vi "RWAE-Fix Name.vi"(8 "error in (no error)":errorcluster, 9 "Section Name (Name of \"Anything\")":string, 10 "Cluster Elements in":variant[](array[variant])) -> (0 "error out":errorcluster, 3 "Name":string)   [LabVIEW 2020]
uses:
  <vilib>/Utility/Data Type/NI_Data Type.lvlib
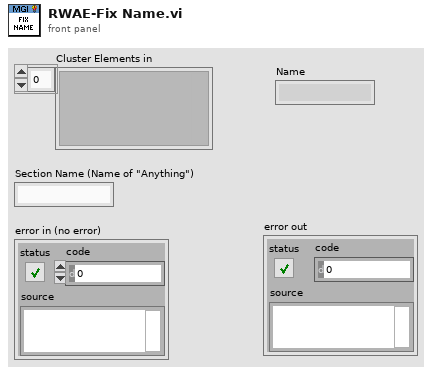
[diagram p1: front panel]
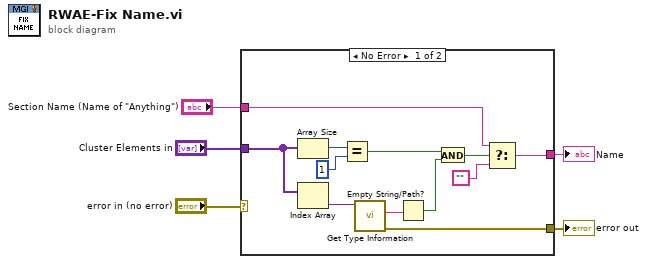
[diagram p0: block diagram]
diagram:
  n1 = case shown="No Error" "error in (no error)" {
    selector: "error in (no error)" -> [_ w18]
    tunnel: "Cluster Elements in" -> [w12 _]
    tunnel: "Section Name (Name of \"Anything\")" -> [w8 _]
    tunnel: [w7 _] -> w2
    tunnel: [w6 w18] -> w1
    frame No Error {
      n2 = Array Size(array=w12) -> (size(s)=w17:i32)
      n3 = Index Array(array=w12) -> (element=w11:variant)  [unwired: 1 in]
      n4 = Equal?(x=w17, y=1) -> (x = y?=w14:bool)
      n5 = call <vilib>:"Get Type Information.vi"("variant"=w11) -> ("error out"=w6:errorcluster, "name"=w15:string)  [unwired: 6 in, 3 out]
      n6 = Empty String/Path?(string/path=w15) -> (empty?=w13:bool)
      n7 = And(x=w14, y=w13) -> (x .and. y?=w10:bool)
      n8 = Select(t=w8, s=w10, f="") -> (s? t:f=w7:string)
    }
    frame Error {
    }
  }
  "Name" <- w2
  "error out" <- w1
